vi "TIFFStream Test.vi"() -> ()   [LabVIEW 2015]
panel:
  in  "Width x Height":i32[](array[numeric])=[2048, 1536]
  out "Current frame":i32
  in  "Print frame numbers?":bool
  in  "File path":path
  in  "Frames":i32=1 min=1
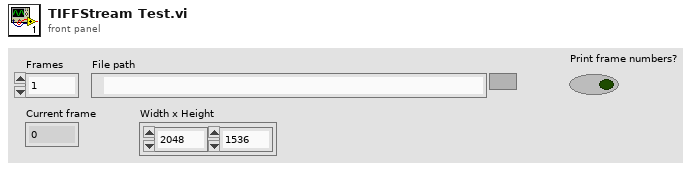
[diagram p1: front panel]
types:
  T1 = cluster{"File refnum":refnum<file>, "Image File Directory":cluster{cluster{"Field":u16, "Type":u16, "Count":u32, "Value / Offset":u32, "Add IFD Offset?":bool}[], cluster{"Data":u32[], "Add offset?":bool}[]}, "Big endian?":bool, "IFD Offset Size":u32}
  T2 = typedef "imagedata.ctl" = cluster{"image type":i32, "image depth":i32, "image":u8[], "mask":u8[], "colors":u32[], "Rectangle":cluster{"left":i16, "top":i16, "right":i16, "bottom":i16}}
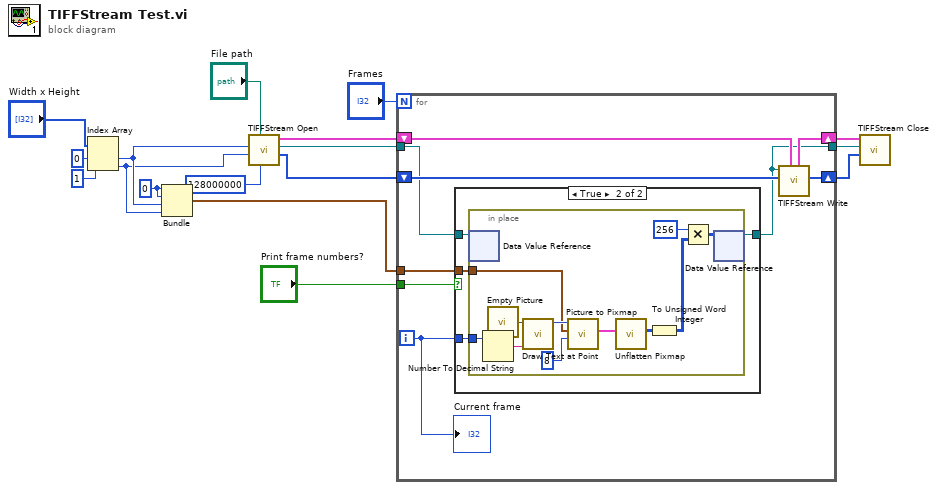
[diagram p0: block diagram]
diagram:
  w5 = 0 ("index")
  n1 = Index Array(array="Width x Height", index #1=0 ("index"), index #2=1 ("index")) -> (element #1=w3:i32, element #2=w2:i32)
  n2 = Bundle("index"=w5, "index"=w5, w3, w2) -> (w4:cluster{"index":i32, "index":i32, i32, i32})  [unwired: 1 in]
  n3 = call "TIFFStream Open.vi"("Bytes per strip"=u32 128000000, "File path"="File path", "Height Pixels"=w2, "Width Pixels"=w3) -> ("Current and next IFD offset"=w13:u32[], "Image data reference"=w15:refnum<data-value>, "File data"=w17:T1)  [unwired: 4 in, 1 out]
  n4 = for {
    N: "Frames" -> [_]
    shift-right: [w25] -> w16
    shift-left: w17 -> [w26]
    tunnel: w15 -> [w22]
    tunnel: [w21] -> w14
    shift-right: [w23] -> w10
    shift-left: w13 -> [w24]
    tunnel: "Print frame numbers?" -> [w19]
    tunnel: w4 -> [w18]
    i -> [w20]
    n5 = case shown="True" w19 {
      tunnel: w22 -> [w27 w31]
      tunnel: [w27 w30] -> w21
      tunnel: w20 -> [_ w29]
      tunnel: w18 -> [_ w28]
      frame False {
      }
      frame True {
        n6 = in-place {
          in-place-border: w29 -> [w35]
          in-place-border: w28 -> [w32]
          n7 = in-place-dvr #1(w31) -> ()  [unwired: 2 out]
          n8 = Number To Decimal String(number=w35) -> (decimal integer string=w34:string)  [unwired: 1 in]
          n9 = call "Empty Picture"() -> ("empty picture"=w33:picture)
          n10 = call <vilib>:"Draw Text at Point.vi"("text"=w34, "picture"=w33) -> ("new picture"=w38:picture)  [unwired: 8 in, 1 out]
          n11 = call <vilib>:"Picture to Pixmap.vi"("depth"=8, "rect"=w32, "picture"=w38) -> ("image data"=w36:T2)  [unwired: 7 in, 1 out]
          n12 = call <vilib>:"Unflatten Pixmap.vi"("image data"=w36) -> ("8-bit pixmap"=w42:u8[][])  [unwired: 4 in, 6 out]
          n13 = To Unsigned Word Integer(number=w42) -> (unsigned 16bit integer=w40:u16[][])
          n14 = Multiply(x=u16 256, y=w40) -> (x*y=w41:u16[][])
          n15 = in-place-dvr #1(w41) -> (w30:refnum<data-value>)  [unwired: 1 out]
        }
      }
    }
    n16 = call "TIFFStream Write.vi"("File data"=w26, "Current and next IFD offset in"=w24, "Image data reference"=w21) -> ("Current and next IFD offset out"=w23:u32[], "File data out"=w25:T1)  [unwired: 6 in, 1 out]
    "Current frame" <- w20
  }
  n17 = call "TIFFStream Close.vi"("Current and next IFD offset"=w10, "Image data reference"=w14, "File data"=w16) -> ()  [unwired: 8 in, 1 out]
